vi "GetConfigurationComboBox(SubVI).vi"(11 "Cluster in":refnum<vi>) -> (3 "ComboBox out":refnum<vi>)   [LabVIEW 2017, in "MainFrameLib.lvlib"]
uses:
  MainFrameLib.lvlib
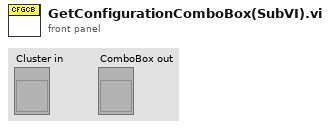
[diagram p1: front panel]
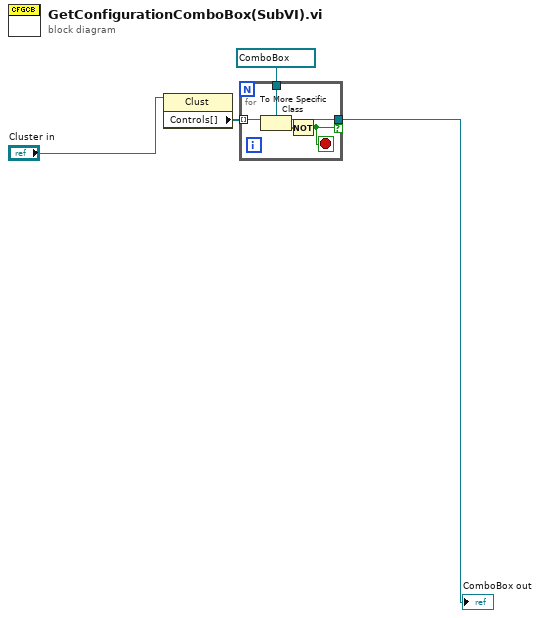
[diagram p0: block diagram]
diagram:
  n1 = property class="Clust"(reference="Cluster in") -> ("Controls[]"=w2:refnum<vi>[])  [unwired: 1 in, 2 out]
  n2 = for {
    tunnel: w2 -> [w8] mode=indexing
    tunnel: refnum<vi> refnum ("Controls.String Controls.Filter AE by Name") -> [w9]
    tunnel: [w6] -> w4 if=w5
    stop <- w5 stop-if-true
    n3 = To More Specific Class(target class=w9, reference=w8) -> (specific class reference=w6:refnum<vi>, error out=w7:errorcluster)  [unwired: 1 in]
    n4 = Not(x=w7) -> (.not. x?=w5:bool)
  }
  "ComboBox out" <- w4
